vi "Msg.vi"(7 "jettl in":refnum<class "jettl.lvclass">, 11 "Event Create Msg Strategy in":refnum<class "Event Create Msg Strategy.lvclass">) -> (5 "jettl out":refnum<class "jettl.lvclass">)   [LabVIEW 2021, in "jettl.lvlib" / "Event Create.lvlib" / "Event Create Msg Strategy.lvclass"]
uses:
  Event Create Msg Strategy.lvclass
  jettl/jettl.lvclass
  Event Create/Event Create.lvclass
  Event Create Msg Strategy.lvclass/Event Create Msg Strategy.ctl
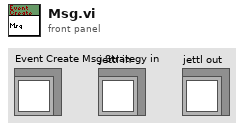
[diagram p1: front panel]
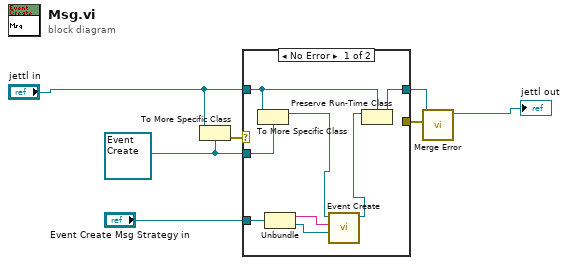
[diagram p0: block diagram]
diagram:
  w1 = refnum<class "Event Create.lvclass"> refnum ("Event Create.lvlib:Event Create.lvclass")
  n1 = To More Specific Class(target class=w1, reference="jettl in") -> (error out=w7:errorcluster)  [unwired: 1 in, 1 out]
  n2 = case shown="No Error" w7 {
    selector: w7 -> [_ w16]
    tunnel: [w13 w17] -> w5
    tunnel: "jettl in" -> [w14 w17]
    tunnel: w1 -> [w15 _]
    tunnel: [_ w16] -> w6
    tunnel: "Event Create Msg Strategy in" -> [w10 _]
    frame No Error {
      n3 = To More Specific Class(target class=w15, reference=w14) -> (specific class reference=w11:refnum<class "Event Create.lvclass">)  [unwired: 1 in, 1 out]
      n4 = Unbundle(w10) -> (w9:string, w8:refnum<class "Event jettl.lvclass">)
      n5 = call-dynamic "Event Create.vi"("Event jettl"=w8, "Alias"=w9, "Event Create in"=w11) -> ("Event Create out"=w12:refnum<class "Event Create.lvclass">)  [unwired: 8 in]
      n6 = Preserve Run-Time Class(object in=w12, 2:w14) -> (object out=w13:refnum<class "jettl.lvclass">)  [unwired: 1 in, 1 out]
    }
    frame Error {
    }
  }
  n7 = call-dynamic "Merge Error.vi"("Error"=w6, "Merge Error in"=w5) -> ("Merge Error out"=→"jettl out":refnum<class "jettl.lvclass">)  [unwired: 9 in]
